vi "Sensor Pcb Gain Cal Eval.vi"(8 "error in (no error)":errorcluster caption="错误输入（无错误）", 9 "numSignals":i32, 10 "sensorSignals":dbl[](array[numeric])=array[4097 elements], 11 "sensorHandle":i32) -> (0 "error out":errorcluster caption="错误输出", 2 "sensorSignals out":dbl[](array[numeric]), 3 "function return":i32)   [LabVIEW 2018]
doc: "extern int __stdcall APSxSensorPcbGainCalEval (int sensorHandle, IN double sensorSignals[], IN int numSignals);"
uses:
  APSx.dll/APSx.dll
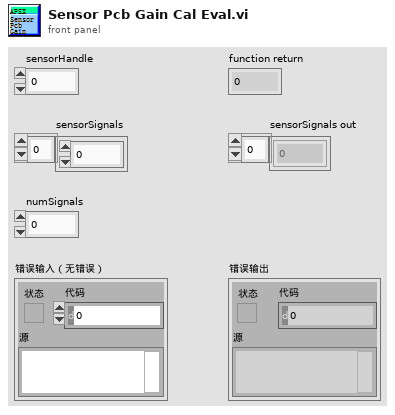
[diagram p1: front panel]
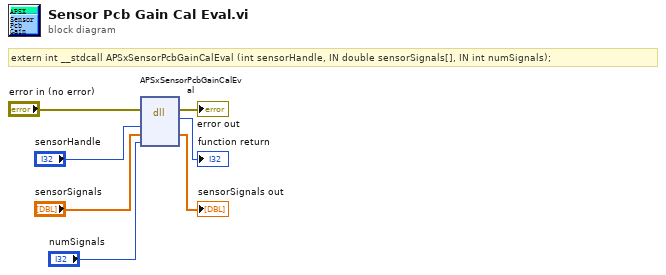
[diagram p0: block diagram]
diagram:
  # "extern int __stdcall APSxSensorPcbGainCalEval (int sensorHandle, IN double sensorSignals[], IN int numSignals);"
  n1 = dll-call lib="PTH2[abs D项目Feng恒隆项目Labview传感器对中台SourcesAPSx.dllAPSx.*" fn="APSxSensorPcbGainCalEval"(error in="error in (no error)", "sensorHandle"="sensorHandle", "sensorSignals"="sensorSignals", "numSignals"="numSignals") -> (error out=→"error out":errorcluster, →"function return":i32, "sensorSignals"=→"sensorSignals out":dbl[])  [unwired: 4 in, 1 out]
